vi "libssh2_userauth_hostbased_fromfile_ex.vi"(4 "local_username":string, 5 "private key":path, 6 "hostname":string, 7 "public key":path, 8 "error in (no error)":errorcluster, 9 "passphrase":string, 10 "username":string, 11 "session":T1) -> (0 "error out":errorcluster)   [LabVIEW 2013, in "libssh2.lvlib"]
doc: "Authenticate a session with a public host key of the client machine, read from file."
uses:
  libssh2.lvlib
  Session Refnum.ctl
  Not A Session.vi
  <vilib>/Utility/error.llb/Error Cluster From Error Code.vi
  Global Settings.vi
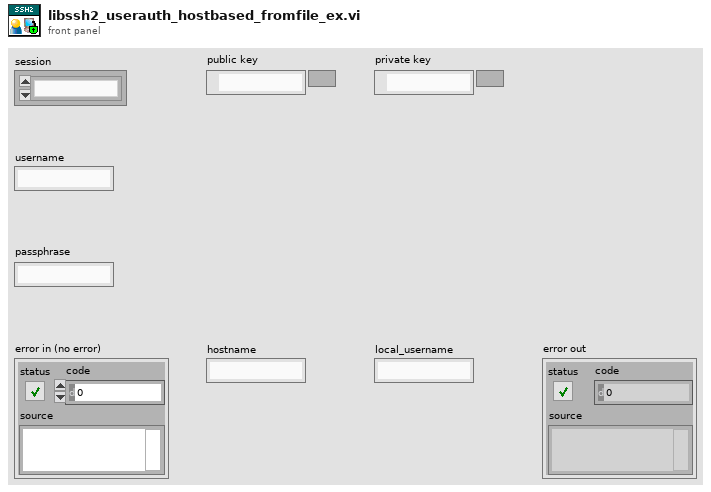
[diagram p1: front panel]
types:
  T1 = typedef "libssh2.lvlib/Session Refnum.ctl" = refnum<k1>
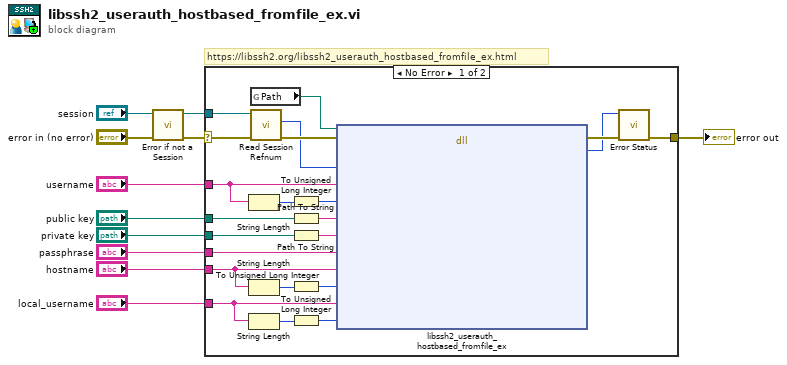
[diagram p0: block diagram]
diagram:
  # "https://libssh2.org/libssh2_userauth_hostbased_fromfile_ex.html"
  n1 = call "Error if not a Session.vi"("error in (no error)"="error in (no error)", "session"="session") -> ("error out"=w8:errorcluster, "session out"=w6:T1)  [unwired: 8 in]
  n2 = case shown="No Error" w8 {
    selector: w8 -> [w32 w34]
    tunnel: "username" -> [w33 _]
    tunnel: [w31 w34] -> w10
    tunnel: w6 -> [w30 _]
    tunnel: "public key" -> [w22 _]
    tunnel: "private key" -> [w21 _]
    tunnel: "passphrase" -> [w20 _]
    tunnel: "hostname" -> [w13 _]
    tunnel: "local_username" -> [w12 _]
    frame No Error {
      n3 = String Length(string=w33) -> (length=w27:i32)
      n4 = String Length(string=w13) -> (length=w17:i32)
      n5 = String Length(string=w12) -> (length=w16:i32)
      n6 = global read "Global Settings.vi" "Path"() -> (w24:path)
      n7 = call "Read Session Refnum.vi"("error in (no error)"=w32, "session"=w30) -> ("error out"=w26:errorcluster, "LIBSSH2_SESSION*"=w25:u64)  [unwired: 5 in, 3 out]
      n8 = To Unsigned Long Integer(number=w27) -> (unsigned 32bit integer=w29:u32)
      n9 = Path To String(path=w22) -> (string=w19:string)
      n10 = Path To String(path=w21) -> (string=w18:string)
      n11 = To Unsigned Long Integer(number=w17) -> (unsigned 32bit integer=w14:u32)
      n12 = To Unsigned Long Integer(number=w16) -> (unsigned 32bit integer=w15:u32)
      n13 = dll-call lib="?" fn="libssh2_userauth_hostbased_fromfile_ex"(path in=w24, error in=w26, "session"=w25, "username"=w33, "username_len"=w29, "publickey"=w19, "privatekey"=w18, "passphrase"=w20, "hostname"=w13, "hostname_len"=w14, "local_username"=w12, "local_username_len"=w15) -> (error out=w28:errorcluster, "return value"=w23:i32)  [unwired: 11 in, 1 out]
      n14 = call "Error Status.vi"("error in (no error)"=w28, "return value"=w23) -> ("error out"=w31:errorcluster)  [unwired: 8 in, 1 out]
    }
    frame Error {
    }
  }
  "error out" <- w10
